vi "Add Data to Circular Buffer.vi"(8 "error in (no error)":errorcluster, 10 "Data":dbl, 11 "Data Plugin in":refnum<class "Data Plugin.lvclass">) -> (0 "error out":errorcluster, 3 "Data Plugin out":refnum<class "Data Plugin.lvclass">)   [LabVIEW 2017, in "Data Engine.lvlib" / "Data Plugin.lvclass"]
uses:
  Data Plugin.lvclass
  Data Plugin.lvclass/Data Plugin.ctl
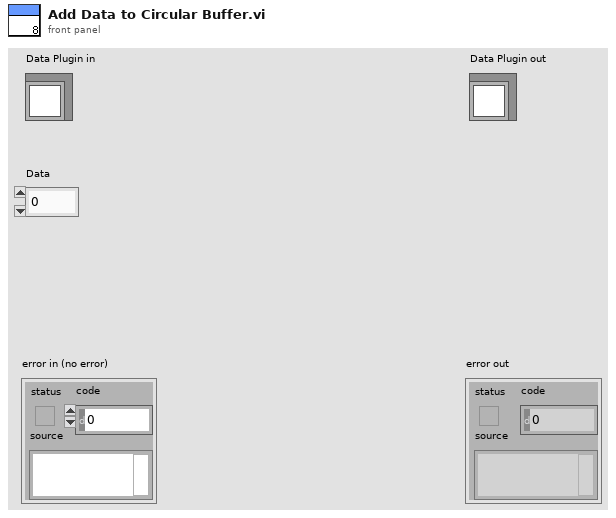
[diagram p1: front panel]
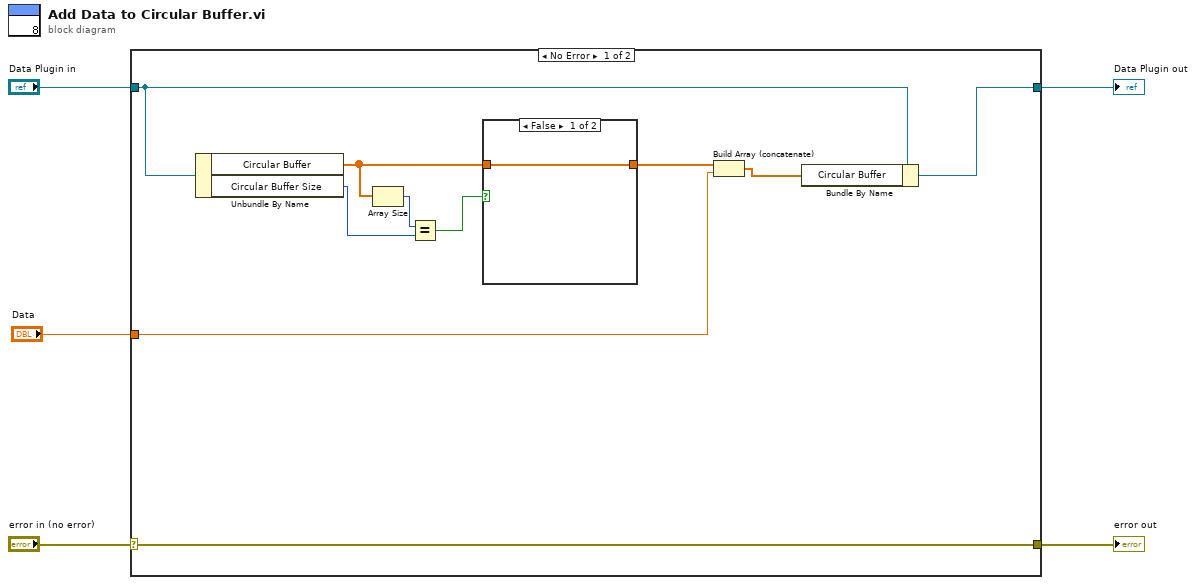
[diagram p0: block diagram]
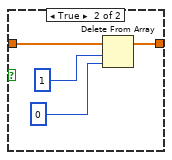
[diagram p2: hidden frame]
diagram:
  n1 = case shown="No Error" "error in (no error)" {
    selector: "error in (no error)" -> [w15 w22]
    tunnel: [w15 w22] -> w4
    tunnel: [w12 w21] -> w2
    tunnel: "Data Plugin in" -> [w14 w21]
    tunnel: "Data" -> [w13 _]
    frame No Error {
      n2 = Unbundle By Name(w14) -> ("Circular Buffer"=w11:dbl[], "Circular Buffer Size"=w6:i32)
      n3 = Array Size(array=w11) -> (size(s)=w10:i32)
      n4 = Equal?(x=w10, y=w6) -> (x = y?=w9:bool)
      n5 = case shown="False" w9 {
        tunnel: w11 -> [w16 w20]
        tunnel: [w16 w17] -> w8
        frame False {
        }
        frame True {
          n6 = Delete From Array(array=w20, length=1, index=0) -> (array with subset deleted=w17:dbl[])  [unwired: 1 out]
        }
      }
      n7 = Build Array (concatenate)(w8, w13) -> (w7:dbl[])
      n8 = Bundle By Name(cluster=w14, "Circular Buffer"=w7) -> (w12:refnum<class "Data Plugin.lvclass">)
    }
    frame Error {
    }
  }
  "error out" <- w4
  "Data Plugin out" <- w2
